vi "Create Export for ni-labviewcli-vipm-operations.vi"() -> ()   [LabVIEW 2014]
uses:
  <vilib>/National Instruments/NIPM API (Beta)/NIPM_API.lvlib
panel:
  out "error out":errorcluster
  out "Generated package (.nipkg) filepath":path
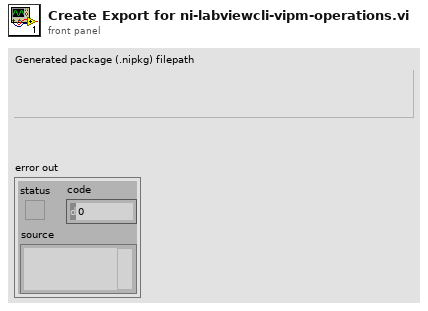
[diagram p1: front panel]
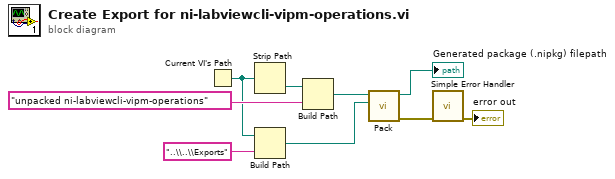
[diagram p0: block diagram]
diagram:
  n1 = Current VI's Path() -> (path=w7:path)
  n2 = Strip Path(path=w7) -> (stripped path=w1:path)  [unwired: 1 out]
  n3 = Build Path(base path=w7, name or relative path="..\\..\\Exports") -> (appended path=w5:path)
  n4 = Build Path(base path=w1, name or relative path="unpacked ni-labviewcli-vipm-operations") -> (appended path=w8:path)
  n5 = call <vilib>:"Pack.vi"("destination folder"=w5, "source folder"=w8) -> ("error out"=w3:errorcluster, "package filepath"=→"Generated package (.nipkg) filepath":path)  [unwired: 8 in]
  n6 = call <vilib>:"Simple Error Handler.vi"("error in (no error)"=w3) -> ("error out"=→"error out":errorcluster)  [unwired: 4 in, 4 out]
